vi "RecognizingEnums.vi"(3 "Array of Cluster with Enum":cluster{"Enum 5":enum16{"c", "d"}}[](array[cluster]), 8 "Cluster With Enum Array":T1, 9 "Cluster With Enum":T2, 10 "Array of Enum":enum16{"c", "d"}[](array[ring]), 11 "Enum":enum16{"c", "d"}(ring)) -> ()   [LabVIEW 2014]
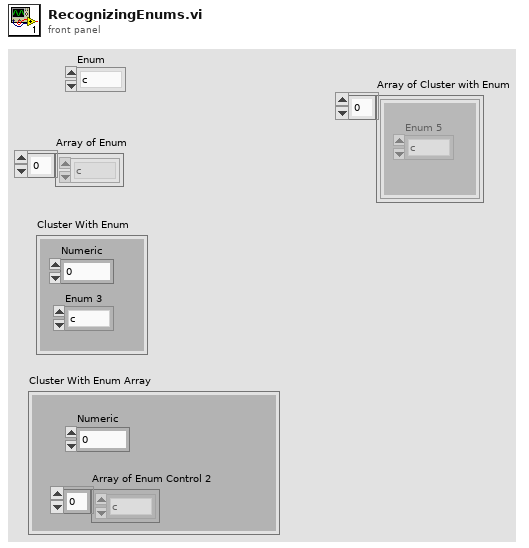
[diagram p1: front panel]
types:
  T1 = cluster{"Array of Enum Control 2":enum16{"c", "d"}[], "Numeric":dbl}
  T2 = cluster{"Enum 3":enum16{"c", "d"}, "Numeric":dbl}
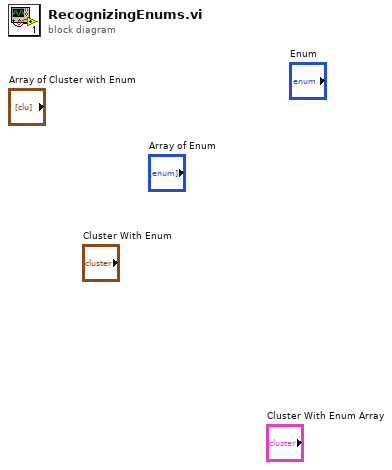
[diagram p0: block diagram]
diagram:
